vi "Write_K7DRAMFIFO.vi"(9 "Input Valid":bool=TRUE, 10 "Element":bool[](array[boolean])=[FALSE, FALSE, FALSE, FALSE, FALSE, FALSE, FALSE, FALSE, FALSE, FALSE, FALSE, FALSE, FALSE, FALSE, FALSE, FALSE, FALSE, FALSE, FALSE, FALSE, FALSE, FALSE, FALSE, FALSE, FALSE, FALSE, FALSE, FALSE, FALSE, FALSE, FALSE, FALSE], 11 "DRAM FIFO Ref In":refnum<class "K7 DRAM FIFO.lvclass">) -> (1 "Ready for Input":bool, 3 "DRAM FIFO Ref Out":refnum<class "K7 DRAM FIFO.lvclass">)   [LabVIEW 2014, in "K7 DRAM FIFO.lvclass"]
doc: "Enqueues a 512 bit boolean array into the DRAM FIFO.\n\n<B>Inputs</B>\n<B>DRAM FIFO Ref In</B> specifies the FIFO. This reference must originate from DRAM FIFO Create.\n<B>Element</B> specifies the 512 bit boolean array data element you want to store in the FIFO.\n<B>Input Valid</B> specifies whether the next data point has arrived for processing. Wire the Output Valid output of an upstream node to this input to transfer data from the upstream node to this node. \n\n<B>Outputs</B>\n<B>DRAM FIFO Ref Out</B> specifies the FIFO. Pass this into DRAM FIFO Read if both write and read are used in the same clock domain.\n<B>Ready for Input</B>returns TRUE if this node is ready to accept new input data. Use a Feedback Node to wire this output to the Ready for Output input of an upstream node. \n\n<B>Detailed Help</B>\nThe Write K7 DRAM FIFO can be used in any clock domain. Note this does not need to be the same clock domain that Read K7 DRAM FIFO resides in, although it can be if desired.\n\nData must first be converted into a boolean array before being passed into Element. If an array of booleans with fewer than 512 elements is passed into Element, the array will be padded withs 0's until it has a width of 512 elements. The Data Manipulation library has functions that assist with converting numeric arrays to boolean arrays.\n\nConsider packing the data before passing it into the FIFO. This prevents the Write k7 DRAM FIFO from overflowing and leads to a more efficient use of DRAM bandwidth. Packing is performed by holding onto data from N previous iterations using a feedback node and 'packing' the data into an array. That array is then submitted to the FIFO every Nth iteration, which reduces the number of elements that are enqueued. The Data Manipulation library has functions that assist with packing.\n\nIf the Ready for Input returns false, the FIFO is full. Consider packing the data. If the FIFO is overflowing after packing the data, try modifying the read/write grant time of the DRAM."
uses:
  K7 DRAM FIFO.lvclass
  K7 DRAM FIFO.lvclass/K7 DRAM FIFO.ctl
  <vilib>/rvi/DataTransferAndStorage/Container/Common/niFpgaContainerExecOnDevCompGetState.vi
  <vilib>/rvi/Emulation/niFpgaEmulationIsFPGAContextNoSignature.vi
  <vilib>/rvi/Emulation/niFpgaSctlEmulationGetInTimedLoop.vi
  <vilib>/rvi/errors/niFpgaSetErrorForExecOnDevCompSimple.vi
  <vilib>/rvi/eio/common/nirviEmuReportErrorAndStop.vi
  <vilib>/rvi/DataTransferAndStorage/Container/Common/niFpgaContainerGetUniqueNameForEmu.vi
  <vilib>/rvi/FIFO/Fifo_Resource/nirvififoEmulationSetSize.vi
  <vilib>/rvi/FIFO/Fifo_Resource/nirviFifoEmulationQueueMgr.vi
  <instcachedir>/0/nirviFifoEmulationQueueMgr_E5CAEC123FF24DC58D834DCA3CDAA9B5.lvgen/nirviFifoEmulationQueueMgr_E5CAEC123FF24DC58D834DCA3CDAA9B5_005.vi
  <vilib>/rvi/FIFO/Fifo_Resource/nirvififoEmulationDetermineInputValidOut.vi
  <vilib>/rvi/FIFO/Fifo_Resource/nirvififoEmulationCreateLock.vi
  <vilib>/rvi/Emulation/niFpgaProcessEmulError.vi
  <vilib>/rvi/FIFO/Fifo_Resource/nirvififoEmulationObtainLock.vi
  <vilib>/rvi/FIFO/Fifo_Resource/nirvififoEmulationReleaseLock.vi
  <vilib>/rvi/occurrence/nirviWaitOnOccurrenceBase.vi
  <vilib>/rvi/errors/nirviReportUnexpectedCaseInternalError.vi
  <vilib>/rvi/errors/nirviReportUnexpectedCaseInternalError (U32).vi
  <vilib>/Utility/error.llb/Clear Errors.vi
  <vilib>/rvi/interface/RandomDataEmulation/niFpgaRandomDataHandleErrors.vi
  <vilib>/rvi/DataTransferAndStorage/Container/XNode/niFpgaContainer.xnode
  <vilib>/rvi/FIFO/Fifo_Resource/niFpgaFifoEmulationRefIn.vi
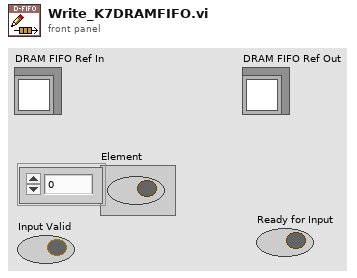
[diagram p1: front panel]
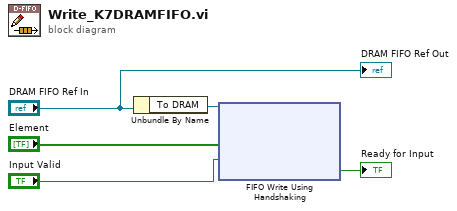
[diagram p0: block diagram]
diagram:
  n1 = Unbundle By Name("DRAM FIFO Ref In") -> ("To DRAM"=w4:refnum<k21>)
  n2 = xnode "FIFO Write Using Handshaking"("Element"="Element", "Input Valid"="Input Valid", "FIFO In"=w4) -> ("Ready for Input"=→"Ready for Input":bool)  [unwired: 1 out]
  "DRAM FIFO Ref Out" <- "DRAM FIFO Ref In"
